vi "实验目录路径.vi"() -> ()   [LabVIEW 2013]
panel:
  in  "实验目录路径":path=path "C:/Users/Xiang MU/Desktop/实验文件夹"
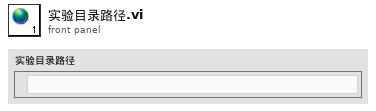
[diagram p1: front panel]
diagram:
